vi "Coder.vi"(11 "Input":string) -> (3 "Output":string)   [LabVIEW 2010, in "DPR250.lvlib"]
uses:
  DPR250.lvlib
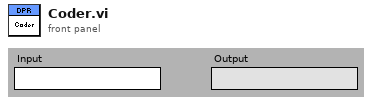
[diagram p1: front panel]
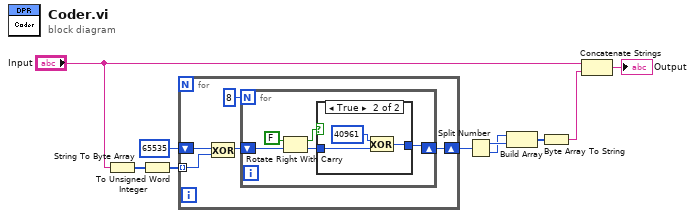
[diagram p0: block diagram]
diagram:
  n1 = String To Byte Array(string="Input") -> (unsigned byte array=w2:u8[])
  n2 = To Unsigned Word Integer(number=w2) -> (unsigned 16bit integer=w3:u16[])
  n3 = for {
    shift-right: [w12] -> w8
    shift-left: u16 65535 -> [w13]
    tunnel: w3 -> [w11] mode=indexing
    n4 = Exclusive Or(1:w11, 2:w13) -> (0:w14:u16)
    n5 = for {
      N: 8 -> [_]
      shift-right: [w19] -> w12
      shift-left: w14 -> [w18]
      n6 = Rotate Right With Carry(2:w18, 3:FALSE ("Übertrag")) -> (0:w20:u16, 1:w17:bool)
      n7 = case shown="True" w17 {
        tunnel: w20 -> [w21 w23]
        tunnel: [w21 w22] -> w19
        frame False {
        }
        frame True {
          n8 = Exclusive Or(1:w23, 2:u16 40961) -> (0:w22:u16)
        }
      }
    }
  }
  n9 = Split Number(x=w8) -> (hi(x)=w7:u8, lo(x)=w6:u8)
  n10 = Build Array(w6, w7) -> (w5:u8[])
  n11 = Byte Array To String(unsigned byte array=w5) -> (string=w9:string)
  n12 = Concatenate Strings("Input", w9) -> (→"Output":string)
